vi "File_Pull data from disc.vi"(8 "Error":errorcluster, 10 "Graphic Root Folder":path, 11 "Data":T1[](array[typedef])) -> (0 "Error Out":errorcluster, 3 "Data Out":T1[](array[typedef]))   [LabVIEW 2021]
uses:
  TypeDefs/Cluster_IconFilename.ctl
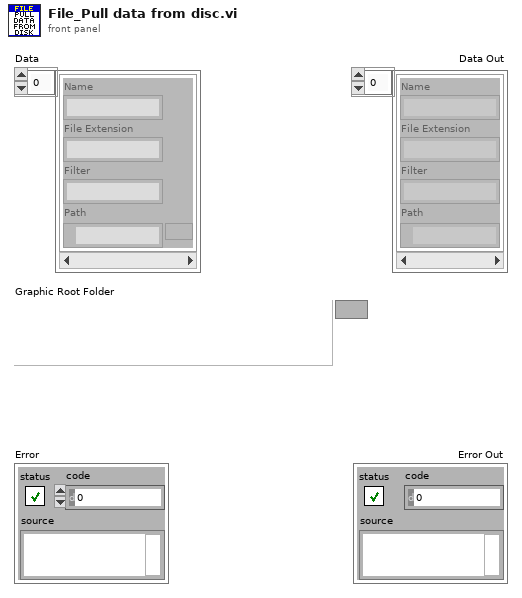
[diagram p1: front panel]
types:
  T1 = typedef "Cluster_IconFilename.ctl" = cluster{"Name":string, "File Extension  ":string, "Filter":string, "Path":path}
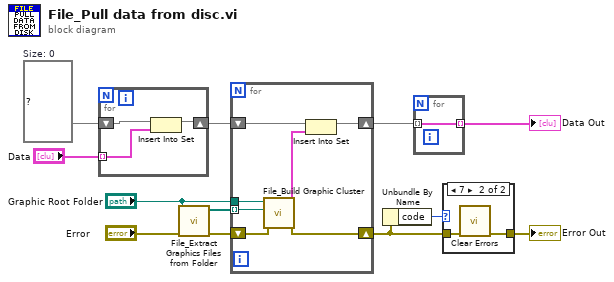
[diagram p0: block diagram]
diagram:
  w4 = set{T1} {}  # Size: 0
  n1 = for {
    tunnel: "Data" -> [w14] mode=indexing
    shift-right: [w13] -> w3
    shift-left: w4 -> [w15]
    n2 = Insert Into Set(10:w14, 11:w15) -> (3:w13:set{T1})  [unwired: 1 out]
  }
  n3 = call "File_Extract Graphics Files from Folder.vi"("Error"="Error", "Graphic Root Folder"="Graphic Root Folder") -> ("Error Out"=w12:errorcluster, "Array Out"=w11:path[])  [unwired: 8 in]
  n4 = for {
    tunnel: w11 -> [w19] mode=indexing
    shift-right: [w21] -> w7
    shift-left: w12 -> [w22]
    tunnel: "Graphic Root Folder" -> [w20]
    shift-right: [w16] -> w2
    shift-left: w3 -> [w18]
    n5 = call "File_Build Graphic Cluster.vi"("Error"=w22, "File Path"=w19, "Graphic Root Folder"=w20) -> ("Error Out"=w21:errorcluster, "Cluster Out"=w17:T1)  [unwired: 7 in]
    n6 = Insert Into Set(10:w17, 11:w18) -> (3:w16:set{T1})  [unwired: 1 out]
  }
  n7 = Unbundle By Name(w7) -> ("code"=w8:i32)
  n8 = for {
    tunnel: w2 -> [w23] mode=indexing
    tunnel: [w23] -> w1 mode=indexing
  }
  "Data Out" <- w1
  n9 = case shown="7" w8 {
    tunnel: w7 -> [w24 w26]
    tunnel: [w24 w25] -> w6
    frame 0, Default {
    }
    frame 7 {
      n10 = call <vilib>:"Clear Errors.vi"("error in (no error)"=w26) -> ("error out"=w25:errorcluster)  [unwired: 1 in, 5 out]
    }
  }
  "Error Out" <- w6
